vi "Untitled 1.vi"   [LabVIEW 2009]
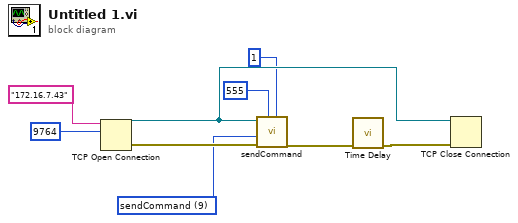
[diagram p0: block diagram]
diagram:
  w3 = u16 9 items=["sendCommand"=9, "FPGA_writeRegister"=3, "FPGA_readRegister"=2, "uC_writeRegister"=1, "uC_readRegister"=0] ("Action")
  n1 = TCP Open Connection(address="172.16.7.43", remote port or service name=u16 9764) -> (connection ID=w6:refnum<k5>, error out=w9:errorcluster)  [unwired: 3 in]
  n2 = call "sendCommand.vi"("number data"=1, "Data"=555, "error in"=w9, "Action"=w3, "connection ID"=w6) -> ("error out"=w8:errorcluster)  [unwired: 2 in, 4 out]
  n3 = call "Time Delay"("error in (no error)"=w8) -> ("error out"=w7:errorcluster)  [unwired: 10 in]
  n4 = TCP Close Connection(connection ID=w6, error in (no error)=w7) -> ()  [unwired: 1 in, 2 out]
